vi "Update Elcom XP.vi"(0 "Run Command":bool, 1 "file path (dialog if empty)":path) -> ()   [LabVIEW 2014]
uses:
  <vilib>/Utility/file.llb/Read From Spreadsheet File (string).vi
  <vilib>/Utility/file.llb/Write To Spreadsheet File (string).vi
panel:
  out "Numeric":i32
  out "subarray":string[](array[string])
  out "Array":string[][](array[string])
  out "subarray 2":string[][](array[string])
  out "all rows":string[][](array[string])
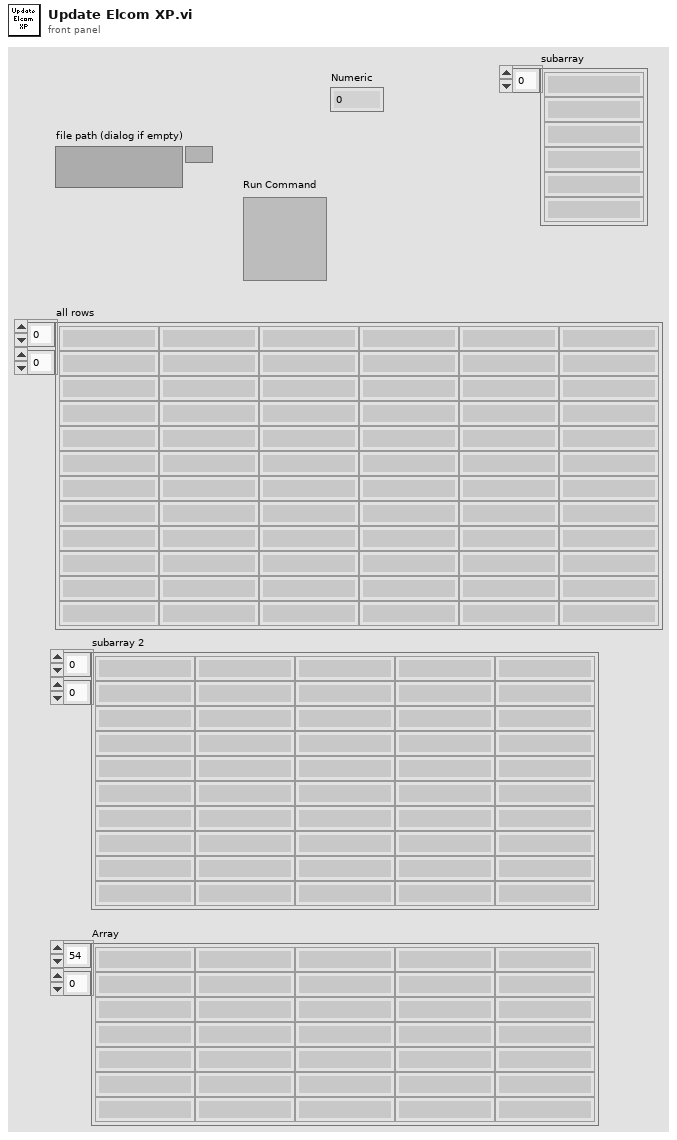
[diagram p1: front panel]
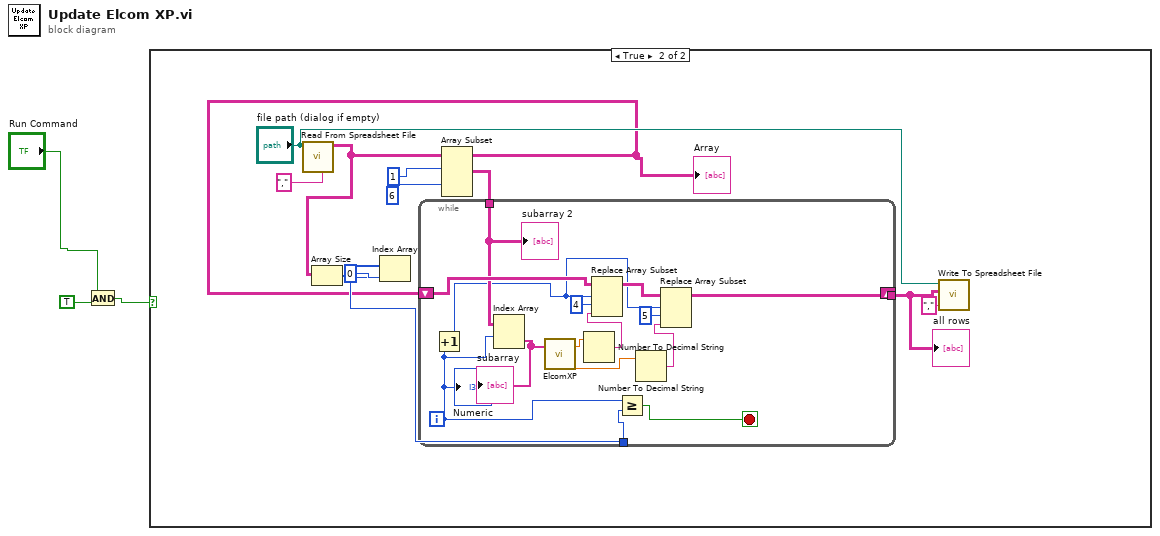
[diagram p0: block diagram]
diagram:
  n1 = And(x="Run Command", y=TRUE) -> (x .and. y?=w3:bool)
  n2 = case shown="True" w3 {
    frame False {
    }
    frame True {
      n3 = call-poly <vilib>:"Read From Spreadsheet File.vi"("delimiter (\\t)"="," ("delimiter (\\t)"), "file path (dialog if empty)"="file path (dialog if empty)") -> ("all rows"=w8:string[][])  [unwired: 5 in, 4 out]
      "Array" <- w8
      n4 = Array Size(array=w8) -> (size(s)=w14:i32[])
      n5 = Index Array(array=w14, index=0) -> (element=w11:i32)
      n6 = Array Subset(array=w8, index (row)=1 ("index"), index (col)=6 ("index")) -> (w5:string[][])  [unwired: 2 in]
      n7 = while {
        tunnel: w11 -> [w29]
        tunnel: [w20] -> w4
        shift-right: [w20] -> _
        shift-left: w8 -> [w19]
        tunnel: w5 -> [w18]
        i -> [w15]
        stop <- w28 stop-if-true
        n8 = Increment(x=w15) -> (x+1=w16:i32)
        n9 = Index Array(array=w18, index (row)=w15) -> (element=w17:string[])  [unwired: 1 in]
        "subarray" <- w17
        n10 = call "ElcomXP.vi"("Input"=w17) -> ("output variable"=w24:dbl, "Elcom XP"=w26:dbl)  [unwired: 1 out]
        n11 = Number To Decimal String(number=w26) -> (decimal integer string=w25:string)  [unwired: 1 in]
        n12 = Replace Array Subset(array=w19, new element=w25, index (row)=w16, index (col)=4 ("disabled index (col)")) -> (w21:string[][])
        n13 = Greater Or Equal?(x=w15, y=w29) -> (x >= y?=w28:bool)
        n14 = Number To Decimal String(number=w24) -> (decimal integer string=w22:string)  [unwired: 1 in]
        n15 = Replace Array Subset(array=w21, new element=w22, index (row)=w16, index (col)=5 ("disabled index (col)")) -> (w20:string[][])
        "subarray 2" <- w18
        "Numeric" <- w15
      }
      "all rows" <- w4
      n16 = call-poly <vilib>:"Write To Spreadsheet File.vi"("delimiter (\\t)"="," ("delimiter (\\t)"), "2D data"=w4, "file path (dialog if empty)"="file path (dialog if empty)") -> ()  [unwired: 5 in, 1 out]
    }
  }
